vi "scale raw data.vi"(9 "channelScaling":T1[](array[typedef]), 10 "raw data":dbl[][](array[numeric]), 11 "scaled data":dbl[][](array[numeric])) -> (3 "scaled data":dbl[][](array[numeric]))   [LabVIEW 2018]
uses:
  PC/type defs/channelControl.ctl
  Type Defs/channelScalingTypes.ctl
  Type Defs/scalingMethods.ctl
  C:/Program Files (x86)/National Instruments/LabVIEW 2018/examples/CompactRIO/Shared/cRIO Convert Thermocouple Readings.llb/Thermocouple Type.ctl
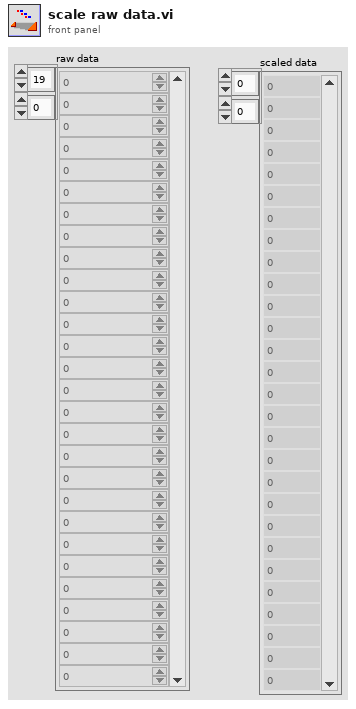
[diagram p1: front panel]
types:
  T1 = typedef "channelControl.ctl" = cluster{"index":u16, "active":bool, "channelType":T2, "module":u16, "terminal":u16, "channelName":string, "scalingMethod":T3, "scalingParameters":dbl[], "scaledUnits":string, "tempOffset":dbl}
  T2 = typedef "channelScalingTypes.ctl" = enum16{"calculation", "measurement", "scanivalve", "output", "digital"}
  T3 = typedef "scalingMethods.ctl" = enum16{"none", "linear", "thermocouple", "polynomial", "encoder", "RTD"}
  T4 = typedef "Thermocouple Type.ctl" = u16
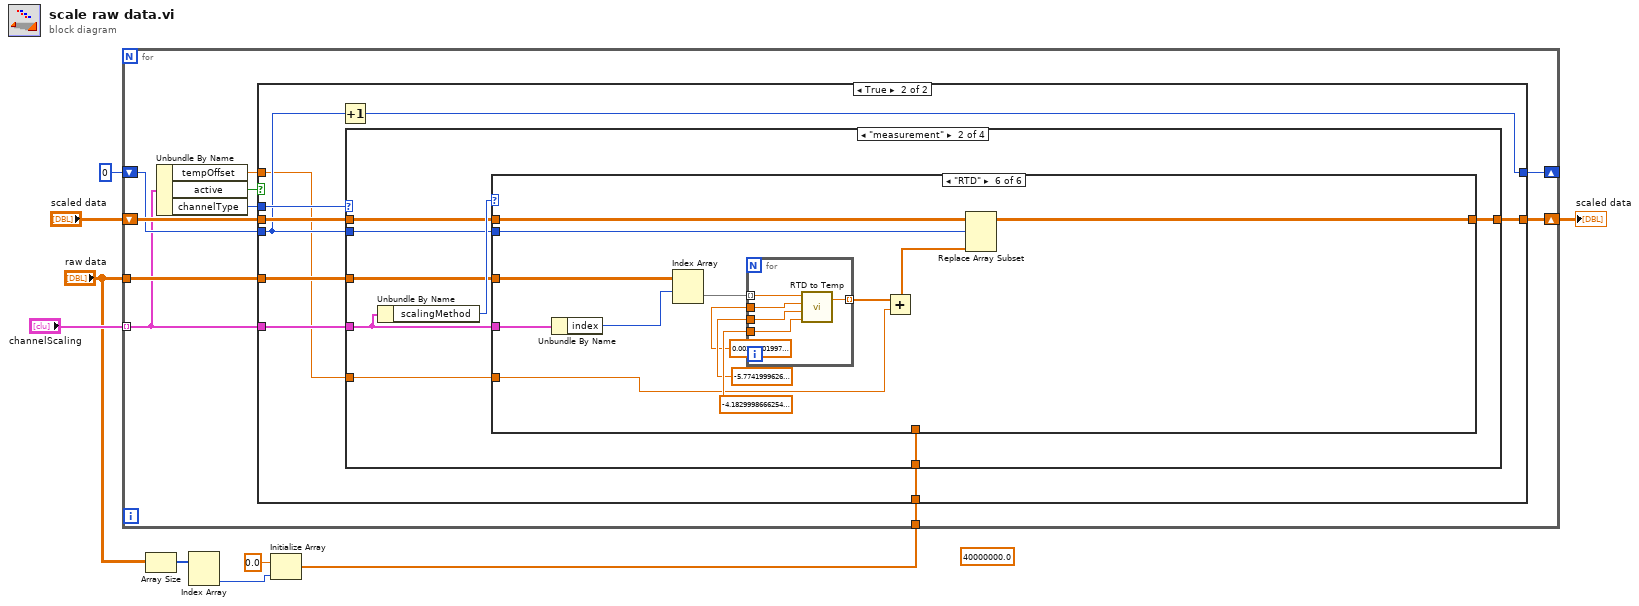
[diagram p0: block diagram]
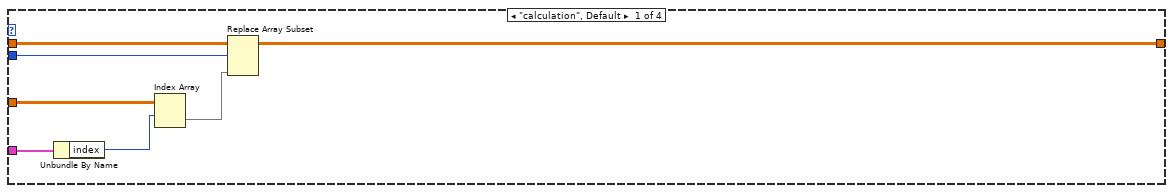
[diagram p3: hidden frame]
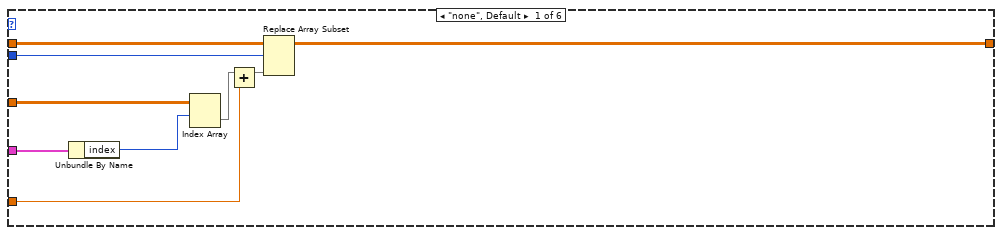
[diagram p4: hidden frame]
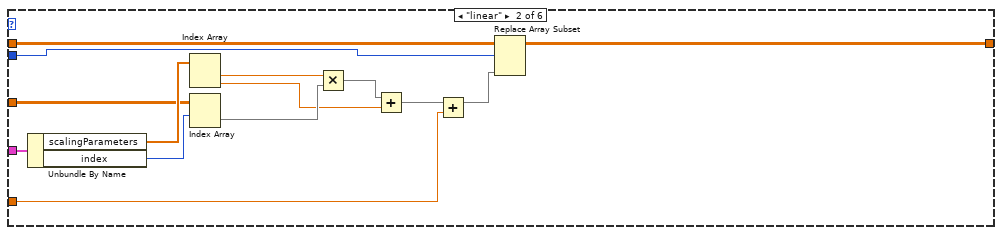
[diagram p5: hidden frame]
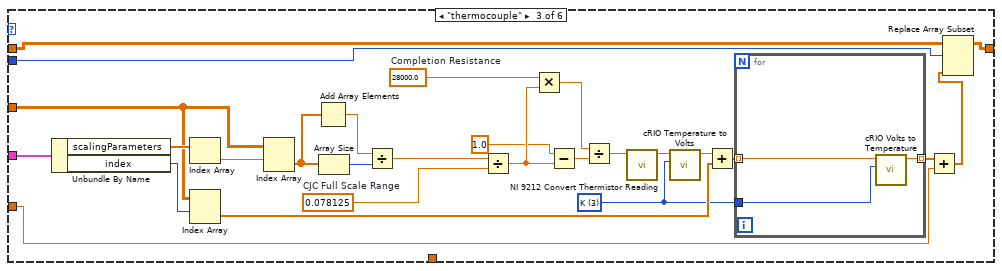
[diagram p6: hidden frame]
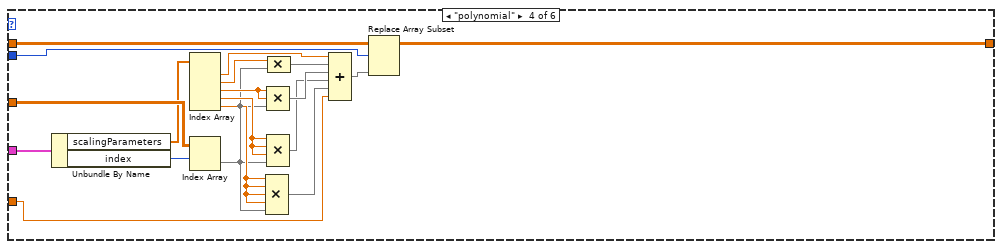
[diagram p7: hidden frame]
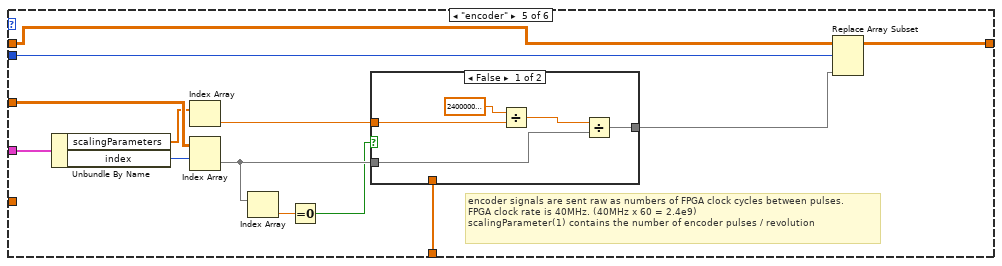
[diagram p8: hidden frame]
diagram:
  (unwired) 40000000.0 ("y")
  n1 = Array Size(array="raw data") -> (size(s)=w3:i32[])
  n2 = Index Array(array=w3) -> (element #2=w2:i32)  [unwired: 2 in, 1 out]
  n3 = Initialize Array(0.0 ("element"), w2) -> (w1:dbl[])
  n4 = for {
    tunnel: "raw data" -> [w13]
    tunnel: "channelScaling" -> [w12] mode=indexing
    shift-right: [w17] -> w8
    shift-left: "scaled data" -> [w18]
    shift-right: [w15] -> _
    shift-left: 0 -> [w14]
    tunnel: w1 -> [w10]
    n5 = Unbundle By Name(w12) -> ("tempOffset"=w11:dbl, "active"=w19:bool, "channelType"=w16:T2)
    n6 = case shown="True" w19 {
      tunnel: w18 -> [w21 w29]
      tunnel: [w21 w26] -> w17
      tunnel: w16 -> [_ w30]
      tunnel: [w20 w24] -> w15
      tunnel: w14 -> [w20 w25]
      tunnel: w13 -> [_ w28]
      tunnel: w12 -> [_ w27]
      tunnel: w11 -> [_ w23]
      tunnel: w10 -> [_ w22]
      frame False {
      }
      frame True {
        n7 = Increment(x=w25) -> (x+1=w24:i32)
        n8 = case shown="\"measurement\"" w30 {
          tunnel: w29 -> [w34 w43 w155 w156]
          tunnel: w25 -> [w33 w41 _ _]
          tunnel: w28 -> [w37 w40 _ _]
          tunnel: w27 -> [w36 w44 _ _]
          tunnel: [w31 w42 w155 w156] -> w26
          tunnel: w23 -> [_ w39 _ _]
          tunnel: w22 -> [_ w38 _ _]
          frame "calculation", Default {
            n9 = Unbundle By Name(w36) -> ("index"=w35:u16)
            n10 = Index Array(array=w37, index (row)=w35) -> (element=w32:dbl[])  [unwired: 1 in]
            n11 = Replace Array Subset(array=w34, new element=w32, index (row)=w33) -> (w31:dbl[][])  [unwired: 1 in]
          }
          frame "measurement" {
            n12 = Unbundle By Name(w44) -> ("scalingMethod"=w45:T3)
            n13 = case shown="\"RTD\"" w45 {
              tunnel: w44 -> [w54 w61 w94 w117 w129 w146]
              tunnel: w43 -> [w53 w68 w95 w113 w130 w142]
              tunnel: [w52 w67 w73 w112 w124 w141] -> w42
              tunnel: w41 -> [w51 w66 w72 w111 w123 w140]
              tunnel: w40 -> [w50 w64 w91 w116 w128 w145]
              tunnel: w39 -> [w46 w55 w69 w99 _ w137]
              tunnel: w38 -> [_ _ _ _ w118 _]
              frame "none", Default {
                n14 = Unbundle By Name(w54) -> ("index"=w49:u16)
                n15 = Index Array(array=w50, index (row)=w49) -> (element=w48:dbl[])  [unwired: 1 in]
                n16 = Add(x=w48, y=w46) -> (x+y=w47:dbl[])
                n17 = Replace Array Subset(array=w53, new element=w47, index (row)=w51) -> (w52:dbl[][])  [unwired: 1 in]
              }
              frame "linear" {
                n18 = Unbundle By Name(w61) -> ("scalingParameters"=w65:dbl[], "index"=w63:u16)
                n19 = Index Array(array=w65) -> (element #1=w62:dbl, element #2=w58:dbl)  [unwired: 2 in]
                n20 = Index Array(array=w64, index (row)=w63) -> (element=w60:dbl[])  [unwired: 1 in]
                n21 = Multiply(x=w62, y=w60) -> (x*y=w59:dbl[])
                n22 = Add(x=w59, y=w58) -> (x+y=w56:dbl[])
                n23 = Add(x=w56, y=w55) -> (x+y=w57:dbl[])
                n24 = Replace Array Subset(array=w68, new element=w57, index (row)=w66) -> (w67:dbl[][])  [unwired: 1 in]
              }
              frame "thermocouple" {
                w74 = T4 3 items=["B", "E", "J", "K", "R", "S", "T", "N"] ("ThermocoupleType")
                w84 = sgl 28000.0  # Completion Resistance
                w85 = sgl 0.078125  # CJC Full Scale Range
                n25 = Unbundle By Name(w94) -> ("scalingParameters"=w93:dbl[], "index"=w92:u16)
                n26 = Index Array(array=w93) -> (element=w90:dbl)  [unwired: 1 in]
                n27 = Index Array(array=w91, index (row)=w92) -> (element=w76:dbl[])  [unwired: 1 in]
                n28 = Index Array(array=w91, index (row)=w90) -> (element=w88:dbl[])  [unwired: 1 in]
                n29 = Add Array Elements(numeric array=w88) -> (sum=w89:dbl)
                n30 = Array Size(array=w88) -> (size(s)=w87:i32)
                n31 = Divide(x=w89, y=w87) -> (x/y=w86:dbl)
                n32 = Divide(x=w86, y=w85) -> (x/y=w82:dbl)
                n33 = Multiply(x=w84, y=w82) -> (x*y=w83:dbl)
                n34 = Subtract(x=sgl 1.0, y=w82) -> (x-y=w80:dbl)
                n35 = Divide(x=w83, y=w80) -> (x/y=w79:dbl)
                n36 = call "NI 9212 Convert Thermistor Reading.vi"("Rt"=w79) -> ("CJC Temperature"=w78:sgl)  [unwired: 10 in]
                n37 = call "cRIO Temperature to Volts.vi"("ThermocoupleType"=w74, "Temperature"=w78) -> ("Thermocouple Voltage"=w75:sgl)  [unwired: 2 in, 3 out]
                n38 = Add(x=w75, y=w76) -> (x+y=w77:dbl[])
                n39 = for {
                  tunnel: w77 -> [w98] mode=indexing
                  tunnel: [w97] -> w71 mode=indexing
                  tunnel: w74 -> [w96]
                  n40 = call "cRIO Volts to Temperature.vi"("ThermocoupleType"=w96, "Thermocouple Voltage"=w98) -> ("Temperature"=w97:sgl)  [unwired: 2 in, 3 out]
                }
                n41 = Add(x=w71, y=w69) -> (x+y=w70:dbl[])
                n42 = Replace Array Subset(array=w95, new element=w70, index (row)=w72) -> (w73:dbl[][])  [unwired: 1 in]
              }
              frame "polynomial" {
                n43 = Unbundle By Name(w117) -> ("scalingParameters"=w114:dbl[], "index"=w115:u16)
                n44 = Index Array(array=w114) -> (element #1=w110:dbl, element #2=w109:dbl, element #3=w107:dbl, element #4=w105:dbl, element #5=w103:dbl)  [unwired: 5 in]
                n45 = Index Array(array=w116, index (row)=w115) -> (element=w102:dbl[])  [unwired: 1 in]
                n46 = Compound Arithmetic op=MULTIPLY(w103, w103, w103, w103, w102) -> (w101:dbl[])
                n47 = Compound Arithmetic op=MULTIPLY(w107, w107, w102) -> (w106:dbl[])
                n48 = Compound Arithmetic op=MULTIPLY(w105, w105, w105, w102) -> (w104:dbl[])
                n49 = Compound Arithmetic op=MULTIPLY(w109, w102) -> (w108:dbl[])
                n50 = Compound Arithmetic op=ADD(w110, w108, w106, w104, w101, w99) -> (w100:dbl[])
                n51 = Replace Array Subset(array=w113, new element=w100, index (row)=w111) -> (w112:dbl[][])  [unwired: 1 in]
              }
              frame "encoder" {
                # "encoder signals are sent raw as numbers of FPGA clock cycles between pulses.\nFPGA clock rate is 40MHz. (40MHz x 60 = 2.4e9)\nscalingParameter(1) contains the number of encoder pulses / revolution"
                n52 = Unbundle By Name(w129) -> ("scalingParameters"=w126:dbl[], "index"=w127:u16)
                n53 = Index Array(array=w126) -> (element=w125:dbl)  [unwired: 1 in]
                n54 = Index Array(array=w128, index (row)=w127) -> (element=w121:dbl[])  [unwired: 1 in]
                n55 = Index Array(array=w121) -> (element=w120:dbl)  [unwired: 1 in]
                n56 = Equal To 0?(x=w120) -> (x = 0?=w119:bool)
                n57 = case shown="False" w119 {
                  tunnel: w125 -> [w134 _]
                  tunnel: [w133 w136] -> w122
                  tunnel: w121 -> [w131 _]
                  tunnel: w118 -> [_ w136]
                  frame False {
                    n58 = Divide(x=2400000000.0 ("Numeric"), y=w134) -> (x/y=w132:dbl)
                    n59 = Divide(x=w132, y=w131) -> (x/y=w133:dbl[])
                  }
                  frame True {
                    # "encoder signal = 0 when motor is not turning"
                  }
                }
                n60 = Replace Array Subset(array=w130, new element=w122, index (row)=w123) -> (w124:dbl[][])  [unwired: 1 in]
              }
              frame "RTD" {
                n61 = Unbundle By Name(w146) -> ("index"=w144:u16)
                n62 = Index Array(array=w145, index (row)=w144) -> (element=w143:dbl[])  [unwired: 1 in]
                n63 = for {
                  tunnel: -4.182999866625403e-12 ("C") -> [w154]
                  tunnel: -5.774199962615967e-07 ("B") -> [w153]
                  tunnel: 0.003908019978553057 ("A") -> [w152]
                  tunnel: w143 -> [w151] mode=indexing
                  tunnel: [w150] -> w139 mode=indexing
                  n64 = call "RTD to Temp.vi"("C"=w154, "B"=w153, "A"=w152, "RTD Resistance"=w151) -> ("RTDtemp"=w150:dbl)  [unwired: 1 out]
                }
                n65 = Add(x=w139, y=w137) -> (x+y=w138:dbl[])
                n66 = Replace Array Subset(array=w142, new element=w138, index (row)=w140) -> (w141:dbl[][])  [unwired: 1 in]
              }
            }
          }
          frame "output" {
          }
          frame "digital" {
          }
        }
      }
    }
  }
  "scaled data" <- w8
